vi "ClosePanel(SubVI).vi"(11 "String":string) -> ()   [LabVIEW 2021]
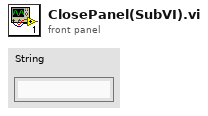
[diagram p1: front panel]
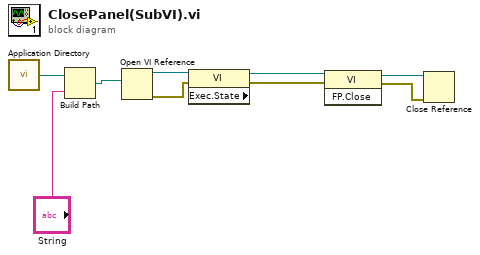
[diagram p0: block diagram]
diagram:
  n1 = call <vilib>:"Application Directory.vi"() -> ("Application Directory"=w8:path)
  n2 = Build Path(base path=w8, name or relative path="String") -> (appended path=w7:path)
  n3 = Open VI Reference(vi path=w7) -> (vi reference=w1:refnum<vi>, error out=w2:errorcluster)  [unwired: 5 in]
  n4 = property class="VI" props=["Exec.State"](reference=w1, error in=w2) -> (reference out=w4:refnum<vi>, error out=w3:errorcluster)  [unwired: 1 out]
  n5 = invoke class="VI" method="FP.Close"(reference=w4, error in=w3) -> (reference out=w5:refnum<vi>, error out=w6:errorcluster)  [unwired: 1 in, 1 out]
  n6 = Close Reference(reference=w5, error in (no error)=w6) -> ()  [unwired: 1 out]
